vi "Unrock_Element_Retrieved.vi"(9 "文件名":string, 10 "路径":path=path "F:/report", 11 "Cluster67":T1) -> ()   [LabVIEW 2019]
uses:
  Unrock_Data.ctl
  <vilib>/Utility/NIReport.llb/Report Type.ctl
  <vilib>/addons/_office/word.llb/Word Find & Replace (str).vi
  <vilib>/Utility/NIReport.llb/NI_ReportGenerationCore.lvlib
  <vilib>/Utility/NIReport.llb/NI_report.lvclass
  <vilib>/addons/_office/NI_ReportGenerationToolkit.lvlib
  <vilib>/Utility/NIReport.llb/Word/NI_Word.lvclass
  TEST.lvclass
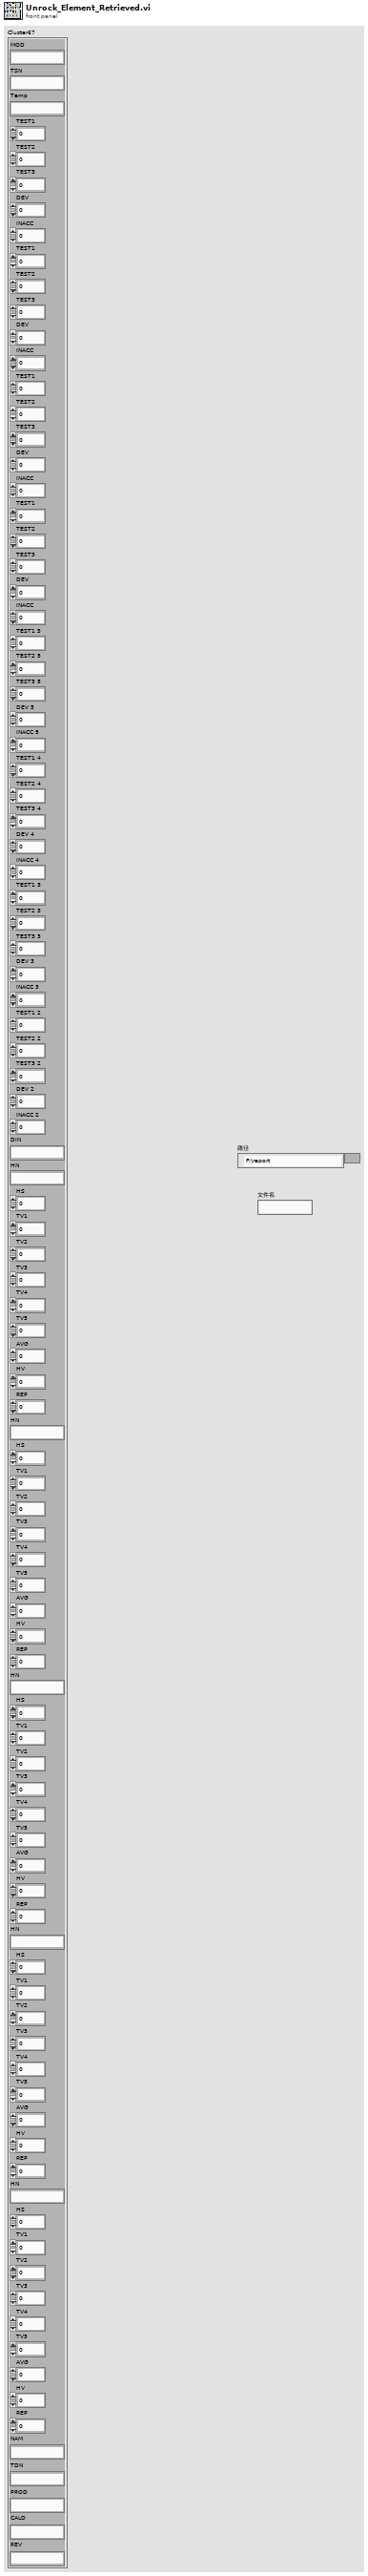
[diagram p1: front panel]
types:
  T1 = typedef "TEST.lvclass/Unrock_Data.ctl" = cluster{"MOD":string, "TSN":string, "Temp":string, "TEST1":sgl, "TEST2":sgl, "TEST3":sgl, "DEV":sgl, "INACC":sgl, "TEST1":sgl, "TEST2":sgl, "TEST3":sgl, "DEV":sgl, "INACC":sgl, "TEST1":sgl, "TEST2":sgl, "TEST3":sgl, "DEV":sgl, "INACC":sgl, "TEST1":sgl, "TEST2":sgl, "TEST3":sgl, "DEV":sgl, "INACC":sgl, "TEST1 5":sgl, "TEST2 5":sgl, "TEST3 5":sgl, "DEV 5":sgl, "INACC 5":sgl, "TEST1 4":sgl, "TEST2 4":sgl, "TEST3 4":sgl, "DEV 4":sgl, "INACC 4":sgl, "TEST1 3":sgl, "TEST2 3":sgl, "TEST3 3":sgl, "DEV 3":sgl, "INACC 3":sgl, "TEST1 2":sgl, "TEST2 2":sgl, "TEST3 2":sgl, "DEV 2":sgl, "INACC 2":sgl, "DIN":string, "HN":string, "HS":sgl, "TV1":sgl, "TV2":sgl, "TV3":sgl, "TV4":sgl, "TV5":sgl, "AVG":sgl, "HV":sgl, "REP":sgl, "HN":string, "HS":sgl, "TV1":sgl, "TV2":sgl, "TV3":sgl, "TV4":sgl, "TV5":sgl, "AVG":sgl, "HV":sgl, "REP":sgl, "HN":string, "HS":sgl, "TV1":sgl, "TV2":sgl, "TV3":sgl, "TV4":sgl, "TV5":sgl, "AVG":sgl, "HV":sgl, "REP":sgl, "HN":string, "HS":sgl, "TV1":sgl, "TV2":sgl, "TV3":sgl, "TV4":sgl, "TV5":sgl, "AVG":sgl, "HV":sgl, "REP":sgl, "HN":string, "HS":sgl, "TV1":sgl, "TV2":sgl, "TV3":sgl, "TV4":sgl, "TV5":sgl, "AVG":sgl, "HV":sgl, "REP":sgl, "NAM":string, "TDN":string, "PROD":string, "CALD":string, "REV":string}
  T2 = typedef "TEST.lvclass/Unrock_Cluster.ctl" = cluster{"MODE":string, "TSN":string, "Temp":string, "Test_load_row1":T3, "Test_load_row2":T3, "Test_load_row3":T3, "Test_load_row4":T3, "Test_load_row5":T3, "Test_load_row6":T3, "Test_load_row7":T3, "Test_load_row8":T3, "DIN":string, "Hardness_test_row1":T4, "Hardness_test_row2":T4, "Hardness_test_row3":T4, "Hardness_test_row4":T4, "Hardness_test_row5":T4}
  T3 = typedef "TEST.lvclass/Test_load.ctl" = cluster{"TEST1":sgl, "TEST2":sgl, "TEST3":sgl, "DEV":sgl, "INACC":sgl}
  T4 = typedef "TEST.lvclass/Hardness_test.ctl" = cluster{"HN":string, "HS":sgl, "TV1":sgl, "TV2":sgl, "TV3":sgl, "TV4":sgl, "TV5":sgl, "AVG":sgl, "HV":sgl, "REP":sgl}
  T5 = typedef "NI_ReportGenerationCore.lvlib/Report Type.ctl" = enum16{"HTML", "Word", "Excel"}
  T6 = enum16{"maximized", "minimized", "normal", "no change"}
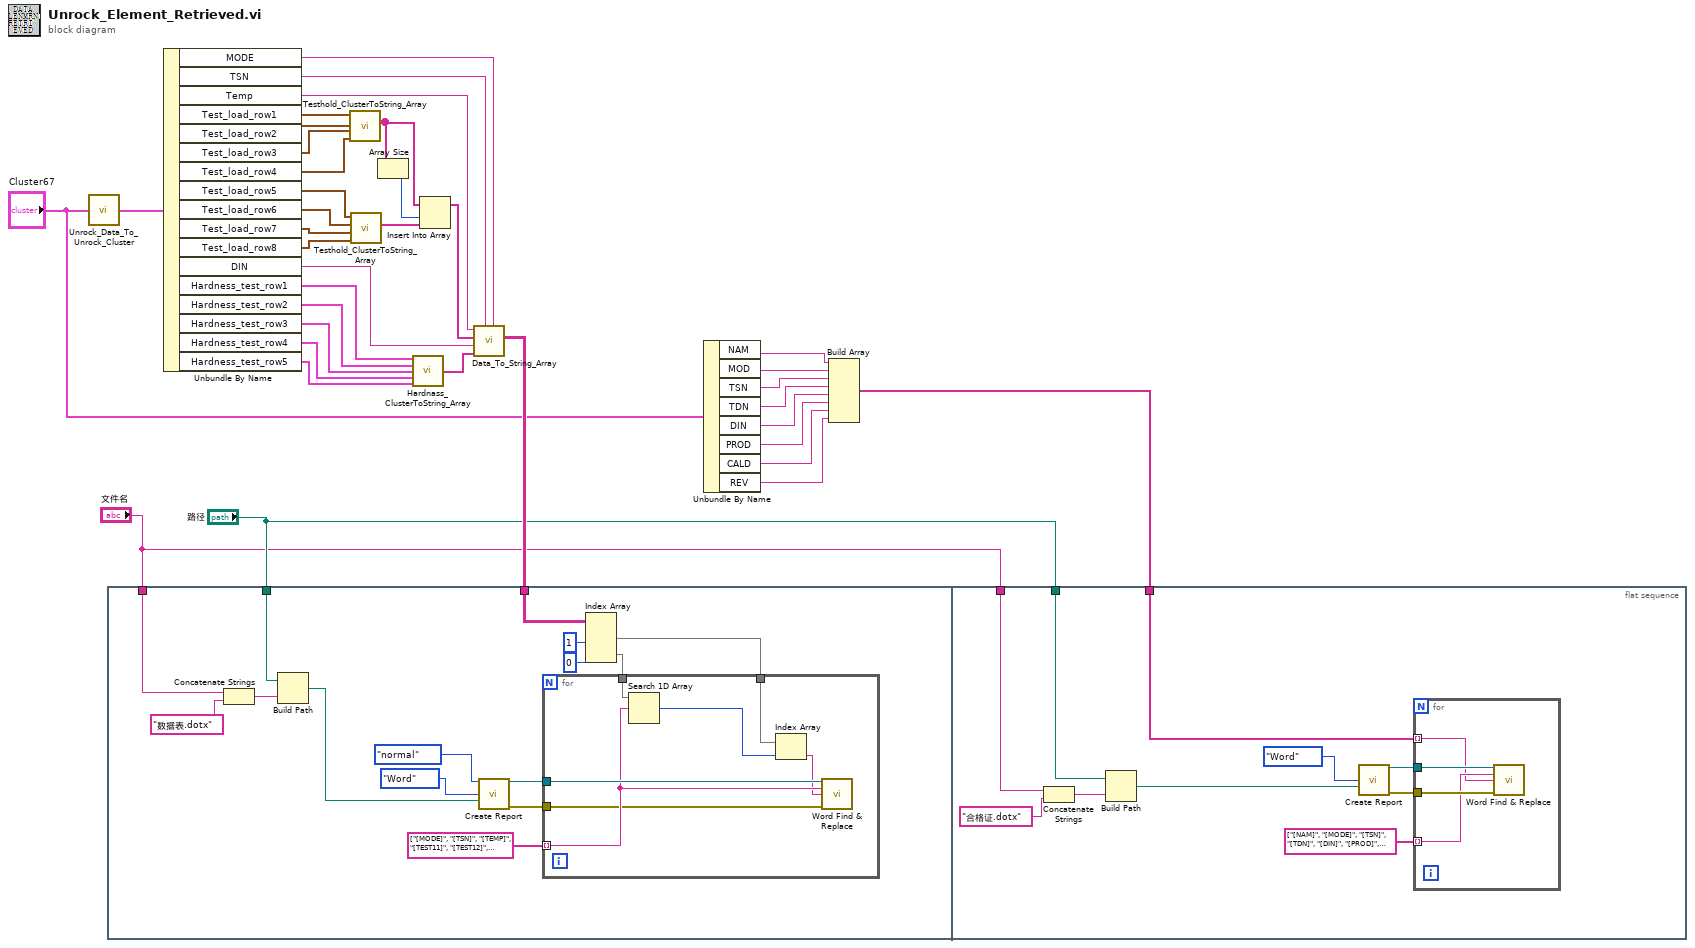
[diagram p0: block diagram]
diagram:
  n1 = call "Unrock_Data_To_Unrock_Cluster.vi"("Cluster67"="Cluster67") -> ("Cluster8"=w32:T2)
  n2 = flat-sequence {
    tunnel: w35 -> [w42]
    tunnel: "路径" -> [w46]
    tunnel: "文件名" -> [w43]
    tunnel: "路径" -> [w61]
    tunnel: "文件名" -> [w60]
    tunnel: w1 -> [w59]
    frame #0 {
      n3 = Concatenate Strings(w43, "数据表.dotx" ("字符串")) -> (w45:string)
      n4 = Build Path(base path=w46, name or relative path=w45) -> (appended path=w47:path)
      n5 = call <vilib>:"Create Report.vi"("window state (normal)"=T6."normal", "report type"=Report_Type."Word", "template (empty)"=w47) -> ("report out"=w49:refnum<class "NI_report.lvclass">, "error out"=w48:errorcluster)  [unwired: 11 in]
      n6 = Index Array(array=w42, index (col) #1=1 ("禁用的索引 (列)"), index (col) #2=0 ("索引 (列)")) -> (element #1=w38:string[], element #2=w39:string[])  [unwired: 2 in]
      n7 = for {
        tunnel: string[] ["[MODE]", "[TSN]", "[TEMP]", "[TEST11]", "[TEST12]", "[TEST13]", "[DEV1]", "[INACC1]", "[TEST21]", "[TEST22]", "[TEST23]", "[DEV2]", "[INACC2]", "[TEST31]", "[TEST32]", "[TEST33]", "[DEV3]", "[INACC3]", "[TEST41]", "[TEST42]", "[TEST43]", "[DEV4]", "[INACC4]", "[TEST51]", "[TEST52]", "[TEST53]", "[DEV5]", "[INACC5]", "[TEST61]", "[TEST62]", "[TEST63]", "[DEV6]", "[INACC6]", "[TEST71]", "[TEST72]", "[TEST73]", "[DEV7]", "[INACC7]", "[TEST81]", "[TEST82]", "[TEST83]", "[DEV8]", "[INACC8]", "[DIN]", "[HN1]", "[HS1]", "[TV11]", "[TV12]", "[TV13]", "[TV14]", "[TV15]", "[AVG1]", "[HV1]", "[REP1]", "[HN2]", "[HS2]", "[TV21]", "[TV22]", "[TV23]", "[TV24]", "[TV25]", "[AVG2]", "[HV2]", "[REP2]", "[HN3]", "[HS3]", "[TV31]", "[TV32]", "[TV33]", "[TV34]", "[TV35]", "[AVG3]", "[HV3]", "[REP3]", "[HN4]", "[HS4]", "[TV41]", "[TV42]", "[TV43]", "[TV44]", "[TV45]", "[AVG4]", "[HV4]", "[REP4]", "[HN5]", "[HS5]", "[TV51]", "[TV52]", "[TV53]", "[TV54]", "[TV55]", "[AVG5]", "[HV5]", "[REP5]"] ("待写入项") -> [w57] mode=indexing
        tunnel: w49 -> [w58]
        tunnel: w48 -> [w56]
        tunnel: w39 -> [w55]
        tunnel: w38 -> [w54]
        n8 = Search 1D Array(1D array=w55, element=w57) -> (index of element=w53:i32)  [unwired: 1 in]
        n9 = Index Array(array=w54, index=w53) -> (element=w52:string)
        n10 = call-poly <vilib>:"Word Find & Replace.vi"("report in"=w58, "find what?"=w57, "replace with"=w52, "error in (no error)"=w56) -> ()  [unwired: 9 in, 3 out]
      }
    }
    frame #1 {
      n11 = Concatenate Strings(w60, "合格证.dotx" ("名称或相对路径")) -> (w64:string)
      n12 = Build Path(base path=w61, name or relative path=w64) -> (appended path=w68:path)
      n13 = call <vilib>:"Create Report.vi"("report type"=Report_Type."Word", "template (empty)"=w68) -> ("report out"=w66:refnum<class "NI_report.lvclass">, "error out"=w65:errorcluster)  [unwired: 12 in]
      n14 = for {
        tunnel: w66 -> [w72]
        tunnel: w65 -> [w71]
        tunnel: string[] ["[NAM]", "[MODE]", "[TSN]", "[TDN]", "[DIN]", "[PROD]", "[CALD]", "[REV]"] ("待写入项 2") -> [w70] mode=indexing
        tunnel: w59 -> [w69] mode=indexing
        n15 = call-poly <vilib>:"Word Find & Replace.vi"("report in"=w72, "find what?"=w70, "replace with"=w69, "error in (no error)"=w71) -> ()  [unwired: 9 in, 3 out]
      }
    }
  }
  n16 = Unbundle By Name(w32) -> ("MODE"=w31:string, "TSN"=w30:string, "Temp"=w29:string, "Test_load_row1"=w23:T3, "Test_load_row2"=w21:T3, "Test_load_row3"=w20:T3, "Test_load_row4"=w19:T3, "Test_load_row5"=w18:T3, "Test_load_row6"=w17:T3, "Test_load_row7"=w16:T3, "Test_load_row8"=w15:T3, "DIN"=w22:string, "Hardness_test_row1"=w28:T4, "Hardness_test_row2"=w27:T4, "Hardness_test_row3"=w26:T4, "Hardness_test_row4"=w25:T4, "Hardness_test_row5"=w24:T4)
  n17 = call "Testhold_ClusterToString_Array.vi"("SLG_Cluster4"=w19, "SLG_Cluster3"=w20, "SLG_Cluster2"=w21, "SLG_Cluster"=w23) -> ("String_Array"=w14:string[])  [unwired: 7 in]
  n18 = call "Testhold_ClusterToString_Array.vi"("SLG_Cluster4"=w15, "SLG_Cluster3"=w16, "SLG_Cluster2"=w17, "SLG_Cluster"=w18) -> ("String_Array"=w12:string[])  [unwired: 7 in]
  n19 = Array Size(array=w14) -> (size(s)=w13:i32)
  n20 = call "Hardnass_ClusterToString_Array.vi"("Hardness_test"=w28, "Hardness_test 2"=w27, "Hardness_test 3"=w26, "Hardness_test 4"=w25, "Hardness_test 5"=w24) -> ("StringArray"=w36:string[])  [unwired: 10 in]
  n21 = Insert Into Array(array=w14, index=w13, new element=w12) -> (w11:string[])
  n22 = call "Data_To_String_Array.vi"("MODE"=w31, "TSN"=w30, "Hardness_string"=w36, "DIN"=w22, "Test_load_string"=w11, "TEMP"=w29) -> ("String_Array"=w35:string[][])  [unwired: 5 in]
  n23 = Unbundle By Name("Cluster67") -> ("NAM"=w9:string, "MOD"=w8:string, "TSN"=w7:string, "TDN"=w6:string, "DIN"=w5:string, "PROD"=w4:string, "CALD"=w3:string, "REV"=w2:string)
  n24 = Build Array(w9, w8, w7, w6, w5, w4, w3, w2) -> (w1:string[])
